vi "Launch BG VI.vi"   [LabVIEW 2020]
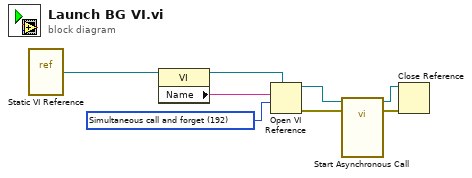
[diagram p0: block diagram]
diagram:
  w6 = 192 items=["Record modifications"=1, "Open templates for editing"=2, "Prompt user to save"=4, "Prepare for reentrant run"=8, "Prompt to find missing subVIs"=16, "Hide loading dialog box"=32, "Enable simultaneous calls"=64, "Prepare to call and forget"=128, "Simultaneous call and forget"=192, "Prepare to call and collect"=256, "Simultaneous call and collect"=320]
  n1 = vi-ref "Static VI Reference"() -> ("vi reference"=w8:refnum<vi>)
  n2 = property class="VI"(reference=w8) -> (reference out=w5:refnum<vi>, "Name"=w7:string)  [unwired: 1 in, 1 out]
  n3 = Open VI Reference(type specifier VI Refnum (for type only)=w5, vi path=w7, options=w6) -> (vi reference=w3:refnum<vi>, error out=w4:errorcluster)  [unwired: 3 in]
  n4 = call-by-ref "Start Asynchronous Call"(reference=w3, error in=w4) -> (reference out=w1:refnum<vi>, error out=w2:errorcluster)
  n5 = Close Reference(reference=w1, error in (no error)=w2) -> ()  [unwired: 1 out]
